vi "getMode.vi"(8 "error in (no error)":errorcluster, 11 "DmmNiPxi in":refnum<class "DmmNi.lvclass">) -> (0 "error out":errorcluster, 2 "mode":T1, 3 "DmmNiPxi out":refnum<class "DmmNi.lvclass">)   [LabVIEW 2023, in "DmmNi.lvclass"]
doc: "<b>Author:</b> Wolfgang\n<b>Description:</b>Query Dmm for measurement mode: Voltage, Current, Resistance"
uses:
  DmmNi.lvclass
  Data/DmmModes.ctl
  DmmNi.lvclass/DmmNi.ctl
  sweDmm.lvlib
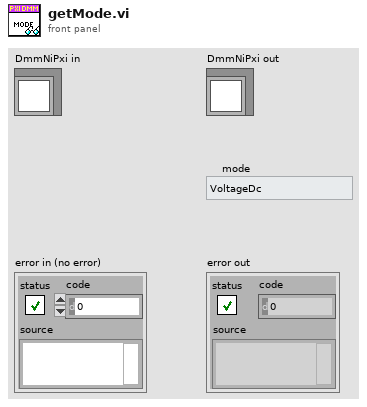
[diagram p1: front panel]
types:
  T1 = typedef "sweDmm.lvlib/DmmModes.ctl" = enum16{"VoltageDc", "VoltageAc", "CurrentDc", "CurrentAc", "Resistance2W"}
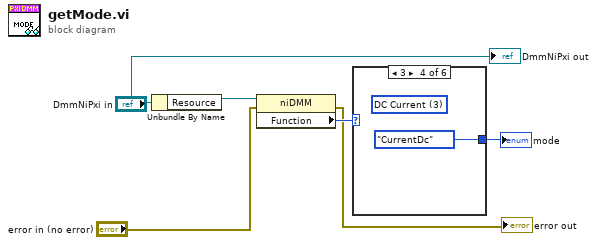
[diagram p0: block diagram]
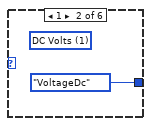
[diagram p3: hidden frame]
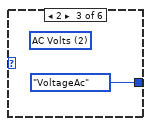
[diagram p4: hidden frame]
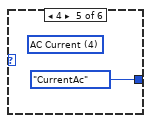
[diagram p5: hidden frame]
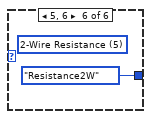
[diagram p6: hidden frame]
diagram:
  n1 = Unbundle By Name("DmmNiPxi in") -> ("Resource"=w6:refnum<k15>)
  n2 = property class="niDMM"(reference=w6, error in="error in (no error)") -> (error out=→"error out":errorcluster, "Function"=w5:i32)  [unwired: 1 out]
  n3 = case shown="3" w5 {
    tunnel: [_ DmmModes."VoltageDc" ("mode") DmmModes."VoltageAc" ("mode") DmmModes."CurrentDc" ("mode") DmmModes."CurrentAc" ("mode") DmmModes."Resistance2W" ("mode")] -> w4
    frame 0, Default {
    }
    frame 1 {
      (unwired) 1 items=["DC Volts"=1, "AC Volts"=2, "DC Current"=3, "AC Current"=4, "2-Wire Resistance"=5, "4-Wire Resistance"=101, "Frequency"=104, "Period"=105, "AC Volts DC Coupled"=1001, "Diode"=1002, "Waveform Voltage"=1003, "Waveform Current"=1004, "Capacitance"=1005, "Inductance"=1006, "Temperature"=108] ("Configuration:Function")
    }
    frame 2 {
      (unwired) 2 items=["DC Volts"=1, "AC Volts"=2, "DC Current"=3, "AC Current"=4, "2-Wire Resistance"=5, "4-Wire Resistance"=101, "Frequency"=104, "Period"=105, "AC Volts DC Coupled"=1001, "Diode"=1002, "Waveform Voltage"=1003, "Waveform Current"=1004, "Capacitance"=1005, "Inductance"=1006, "Temperature"=108] ("Configuration:Function")
    }
    frame 3 {
      (unwired) 3 items=["DC Volts"=1, "AC Volts"=2, "DC Current"=3, "AC Current"=4, "2-Wire Resistance"=5, "4-Wire Resistance"=101, "Frequency"=104, "Period"=105, "AC Volts DC Coupled"=1001, "Diode"=1002, "Waveform Voltage"=1003, "Waveform Current"=1004, "Capacitance"=1005, "Inductance"=1006, "Temperature"=108] ("Configuration:Function")
    }
    frame 4 {
      (unwired) 4 items=["DC Volts"=1, "AC Volts"=2, "DC Current"=3, "AC Current"=4, "2-Wire Resistance"=5, "4-Wire Resistance"=101, "Frequency"=104, "Period"=105, "AC Volts DC Coupled"=1001, "Diode"=1002, "Waveform Voltage"=1003, "Waveform Current"=1004, "Capacitance"=1005, "Inductance"=1006, "Temperature"=108] ("Configuration:Function")
    }
    frame 5, 6 {
      (unwired) 5 items=["DC Volts"=1, "AC Volts"=2, "DC Current"=3, "AC Current"=4, "2-Wire Resistance"=5, "4-Wire Resistance"=101, "Frequency"=104, "Period"=105, "AC Volts DC Coupled"=1001, "Diode"=1002, "Waveform Voltage"=1003, "Waveform Current"=1004, "Capacitance"=1005, "Inductance"=1006, "Temperature"=108] ("Configuration:Function")
    }
  }
  "mode" <- w4
  "DmmNiPxi out" <- "DmmNiPxi in"
